vi "base64-decode.vi"(0 "String":string) -> (1 "binary output":string, 2 "return code":i32)   [LabVIEW 2013]
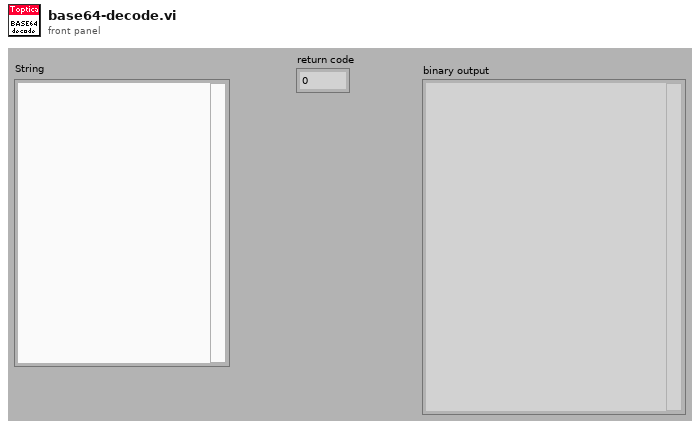
[diagram p1: front panel]
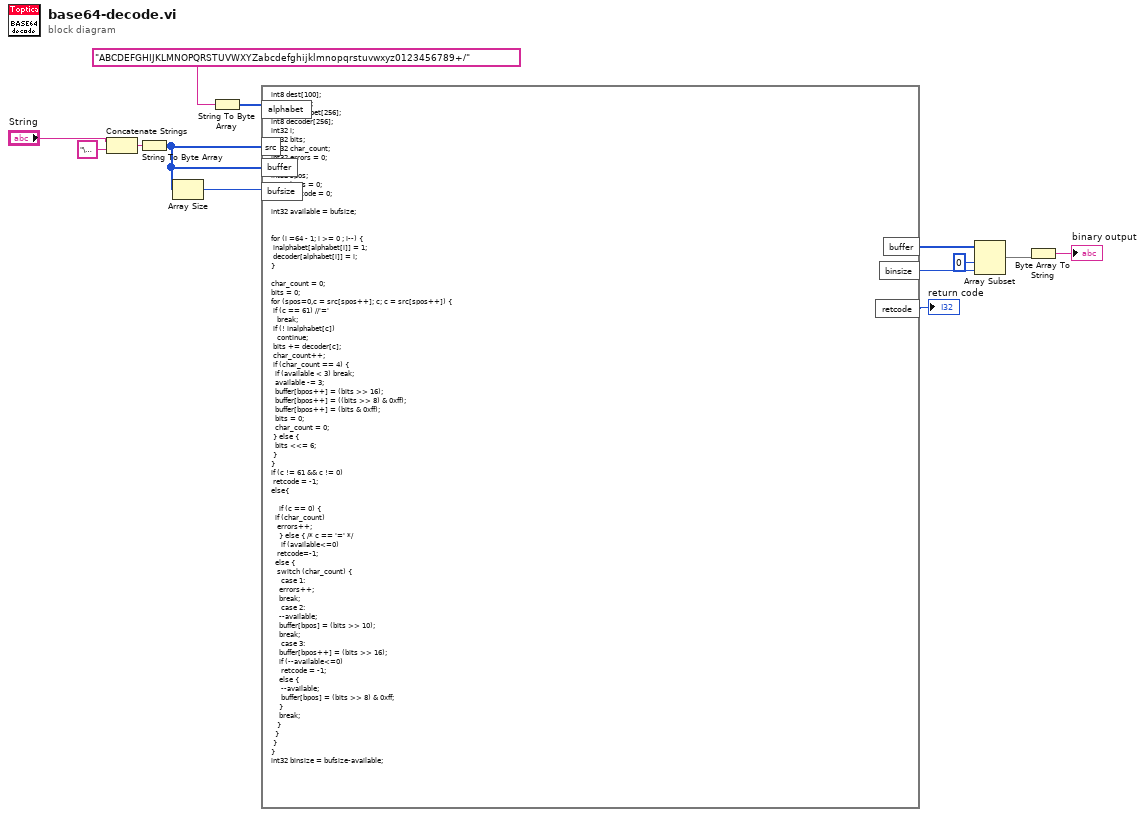
[diagram p0: block diagram]
diagram:
  n1 = Concatenate Strings("String", "\u0000" ("string")) -> (w7:string)
  n2 = String To Byte Array(string=w7) -> (unsigned byte array=w10:u8[])
  n3 = Array Size(array=w10) -> (size(s)=w11:i32)
  n4 = String To Byte Array(string="ABCDEFGHIJKLMNOPQRSTUVWXYZabcdefghijklmnopqrstuvwxyz0123456789+/") -> (unsigned byte array=w13:u8[])
  n5 = formula code="int8 dest[100];\nint destsize;\nint8 inalphabet[256];\nint8 decoder[256];\nint32 i;\nint32 bits;\nint32 char_count;\nint32 errors = 0;\nuInt8 c;\nint32 spos;\nint32 bpos = 0;\nint32 retcode = 0;\n\nint32 available = bufsize;\n\n\nfor (i =64 - 1; i >= 0 ; i--) {\n\tinalphabet[alphabet[i]] = 1;\n\tdecoder[alphabet[i]] = i;\n}\n\nchar_count = 0;\nbits = 0;\nfor (spos=0,c = src[spos++]; c; c = src[spos++]) {\n\tif (c == 61) //'='\n\t  break;\n\tif (! inalphabet[c])\n\t  continue;\n\tbits += decoder[c];\n\tchar_count++;\n\tif (char_count == 4) {\n\t\tif (available < 3) break;\n\t\tavailable -= 3;\n\t\tbuffer[bpos++] = (bits >> 16);\n\t\tbuffer[bpos++] = ((bits >> 8) & 0xff);\n\t\tbuffer[bpos++] = (bits & 0xff);\n\t\tbits = 0;\n\t\tchar_count = 0;\n\t} else {\n\t\tbits <<= 6;\n\t}\n}\nif (c != 61 && c != 0)\n\tretcode = -1;\nelse{\n\n    if (c == 0) {\n\t\tif (char_count)\n\t\t\terrors++;\n    } else { /* c == '=' */\n    \tif (available<=0)\n\t\t\tretcode=-1;\n\t\telse {\n\t\t\tswitch (char_count) {\n\t\t\t  case 1:\n\t\t\t\terrors++;\n\t\t\t\tbreak;\n\t\t\t  case 2:\n\t\t\t\t--available;\n\t\t\t\tbuffer[bpos] = (bits >> 10);\n\t\t\t\tbreak;\n\t\t\t  case 3:\n\t\t\t\tbuffer[bpos++] = (bits >> 16);\n\t\t\t\tif (--available<=0)\n\t\t\t\t\tretcode = -1;\n\t\t\t\telse {\n\t\t\t\t\t--available;\n\t\t\t\t\tbuffer[bpos] = (bits >> 8) & 0xff;\n\t\t\t\t}\n\t\t\t\tbreak;\n\t\t\t}\n\t\t}\n\t}\n}\nint32 binsize = bufsize-available;"("src"=w10, "alphabet"=w13, "bufsize"=w11, "buffer"=w10) -> ("buffer"=w6:u8[], "retcode"=→"return code":i32, "binsize"=w5:i32)
  n6 = Array Subset(array=w6, index=0, length=w5) -> (w2:u8[])
  n7 = Byte Array To String(unsigned byte array=w2) -> (string=→"binary output":string)
